vi "Initialize Value Expression.vi"(8 "error in (no error)":errorcluster, 10 "Expression string":string, 11 "Output Sequencer in":refnum<class "Output Sequencer.lvclass">) -> (0 "error out":errorcluster, 2 "Expression Data":T1, 3 "Output Sequencer out":refnum<class "Output Sequencer.lvclass">)   [LabVIEW 2024, in "Output Sequencer.lvlib" / "Output Sequencer.lvclass"]
uses:
  Output Sequencer.lvclass
  Types/Expression Data.ctl
  <vilib>/LAVA/muParser/mupExpr/mupExpr.lvclass
  Globals/Global Strings.vi
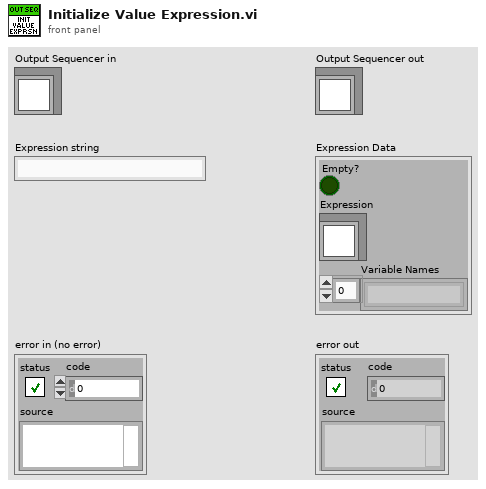
[diagram p1: front panel]
types:
  T1 = typedef "Output Sequencer.lvlib/Output Sequencer.lvclass/Expression Data.ctl" = cluster{"Empty?":bool, "Expression":refnum<class "mupExpr.lvclass">, "Variable Names":string[]}
  T2 = cluster{"error code":i32, "error message":string, "error pos":i32, "error token":string}
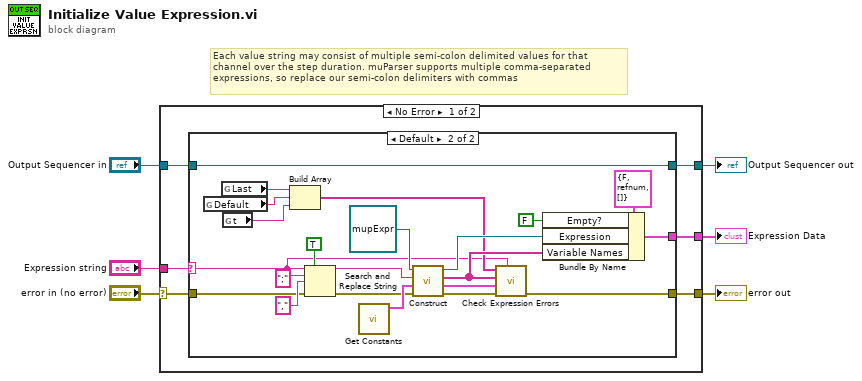
[diagram p0: block diagram]
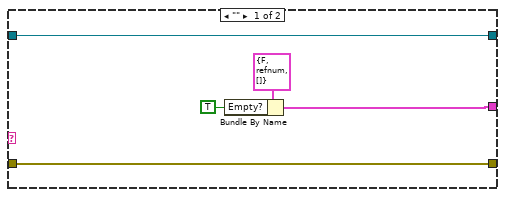
[diagram p2: hidden frame]
diagram:
  # "Each value string may consist of multiple semi-colon delimited values for that\nchannel over the step duration. muParser supports multiple comma-separated\nexpressions, so replace our semi-colon delimiters with commas"
  n1 = case shown="No Error" "error in (no error)" {
    selector: "error in (no error)" -> [w7 w41]
    tunnel: [w12 _] -> w6
    tunnel: "Expression string" -> [w11 _]
    tunnel: [w10 w41] -> w4
    tunnel: "Output Sequencer in" -> [w9 w40]
    tunnel: [w8 w40] -> w2
    frame No Error {
      n2 = case shown="Default" w11 {
        selector: w11 -> [_ w18]
        tunnel: w9 -> [w13 w33]
        tunnel: w7 -> [w14 w25]
        tunnel: [w14 w29] -> w10
        tunnel: [w16 w35] -> w12
        tunnel: [w13 w33] -> w8
        frame "" {
          n3 = Bundle By Name(cluster=T1 {"Empty?"=FALSE, "Expression"=refnum, "Variable Names"=[]} ("Expression Data"), "Empty?"=TRUE) -> (w16:T1)
        }
        frame Default {
          n4 = global read "Global Strings.vi" "Default"() -> (w22:string)
          n5 = global read "Global Strings.vi" "Last"() -> (w20:string)
          n6 = global read "Global Strings.vi" "t"() -> (w21:string)
          n7 = Build Array(w20, w22, w21) -> (w19:string[])
          n8 = Search and Replace String(replace all?=TRUE ("replace all? (F)"), input string=w18, search string=";", replace string="," ("replace string (\"\")"), error in=w25) -> (result string=w23:string, error out=w24:errorcluster)  [unwired: 3 in, 2 out]
          n9 = call "Get Constants.vi"() -> ("Constants"=w36:cluster{"name":string, "value":dbl}[])  [unwired: 11 in]
          n10 = call-dynamic "Construct.vi"("error in (no error)"=w24, "Constants"=w36, "Expression"=w23, "muExpr in"=refnum<class "mupExpr.lvclass"> refnum) -> ("error out"=w32:errorcluster, "error details"=w31:T2, "Variable Names"=w30:string[], "mupExpr out"=w39:refnum<class "mupExpr.lvclass">)  [unwired: 4 in]
          n11 = call "Check Expression Errors.vi"("Expression String in"=w18, "error in (no error)"=w32, "Parser Error Details"=w31, "Found Variables"=w30, "Expected Variables"=w19) -> ("error out"=w29:errorcluster)  [unwired: 6 in]
          n12 = Bundle By Name(cluster=T1 {"Empty?"=FALSE, "Expression"=refnum, "Variable Names"=[]} ("Expression Data"), "Empty?"=FALSE, "Expression"=w39, "Variable Names"=w30) -> (w35:T1)
        }
      }
    }
    frame Error {
    }
  }
  "Expression Data" <- w6
  "error out" <- w4
  "Output Sequencer out" <- w2
